vi "Execute (Multiple result with rows).vi"(8 "error in (no error)":errorcluster, 10 "SQL":string, 11 "PQ Connection in":refnum<class "PQ Connection.lvclass">) -> (0 "error out":errorcluster, 1 "Results with Rows returned":refnum<class "PQ Result.lvclass">[](array[class]), 3 "PQ Connection out":refnum<class "PQ Connection.lvclass">)   [LabVIEW 2016, in "PQ Connection.lvclass"]
uses:
  PQ Connection.lvclass
  Result/PQ Result.lvclass
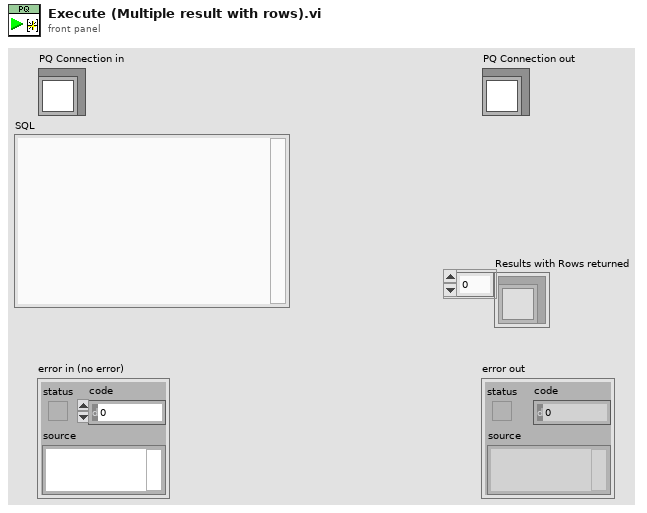
[diagram p1: front panel]
types:
  T1 = typedef "PQ Result.lvclass/Result Status.ctl" = enum32{"PGRES_EMPTY_QUERY", "PGRES_COMMAND_OK", "PGRES_TUPLES_OK", "PGRES_COPY_OUT", "PGRES_COPY_IN", "PGRES_BAD_RESPONSE", "PGRES_NONFATAL_ERROR", "PGRES_FATAL_ERROR", "PGRES_COPY_BOTH", "PGRES_SINGLE_TUPLE"}
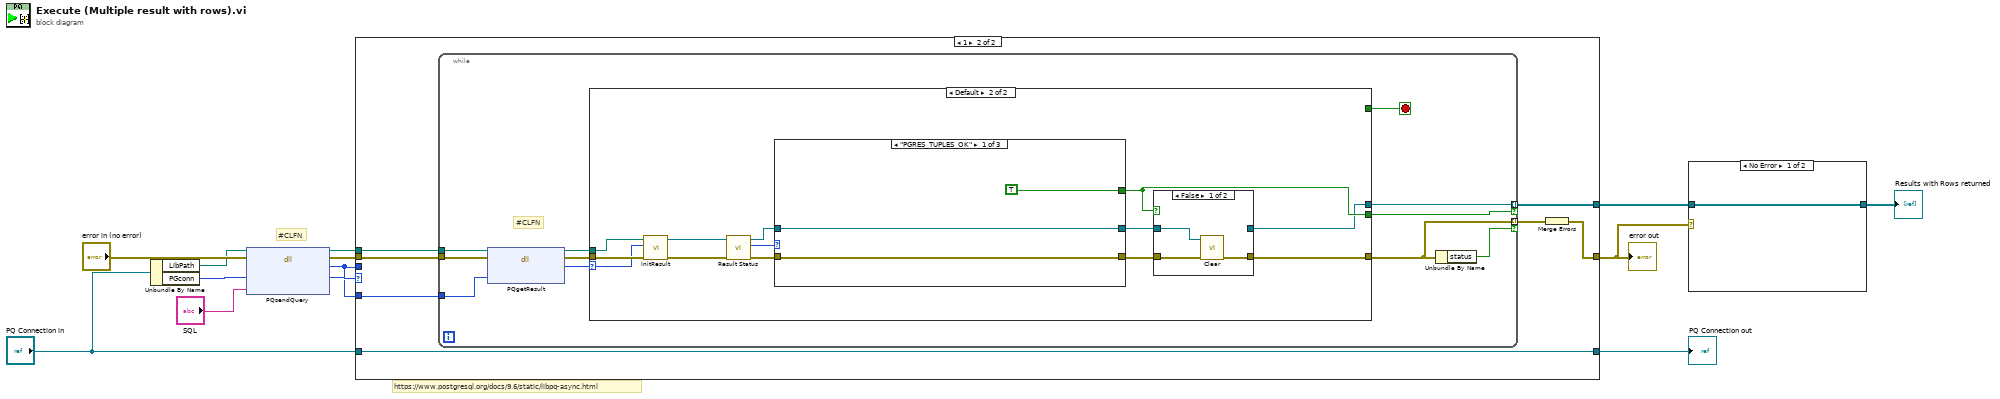
[diagram p0: block diagram]
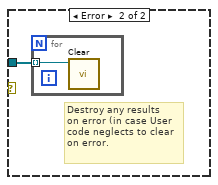
[diagram p2: hidden frame]
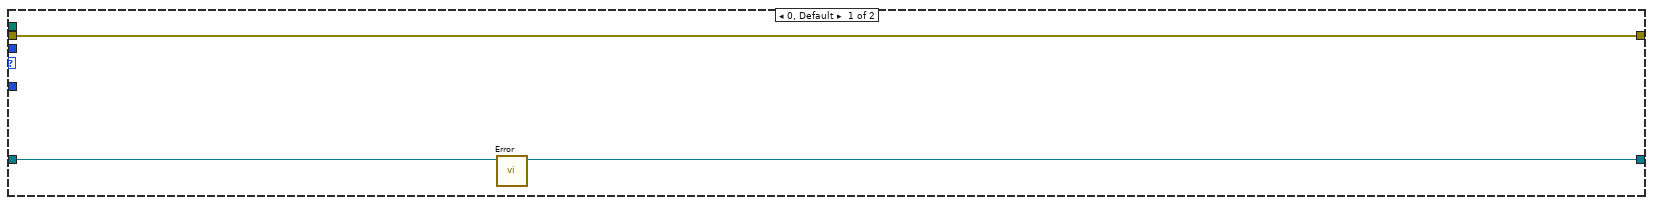
[diagram p3: hidden frame]
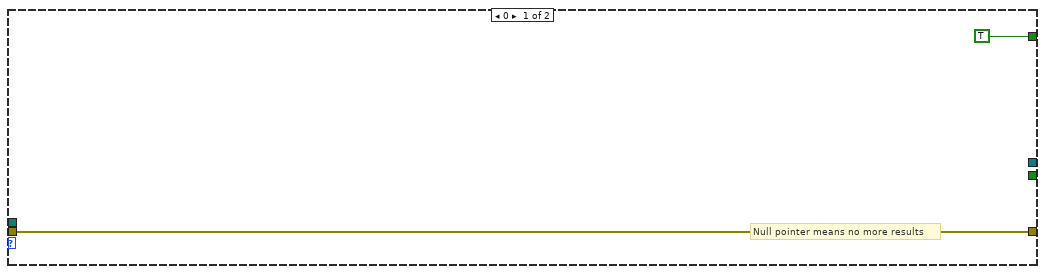
[diagram p4: hidden frame]
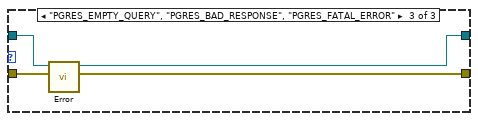
[diagram p6: hidden frame]
diagram:
  # "#CLFN"
  # "https://www.postgresql.org/docs/9.6/static/libpq-async.html"
  n1 = Unbundle By Name("PQ Connection in") -> ("LibPath"=w2:path, "PGconn"=w12:u32)
  n2 = dll-call lib="libpq.*" fn="PQsendQuery" ("libpq.*:PQexec")(path in=w2, error in="error in (no error)", "PGconn"=w12, "command"="SQL") -> (path out=w1:path, error out=w11:errorcluster, "OK?"=w9:u32, "PGconn"=w6:u32)  [unwired: 2 in]
  n3 = case shown="1" w9 {
    tunnel: w11 -> [w14 w23]
    tunnel: w9 -> [_ _]
    tunnel: [_ w22] -> w4
    tunnel: [w14 w18] -> w3
    tunnel: "PQ Connection in" -> [w16 w19]
    tunnel: [w15 w19] -> w7
    tunnel: w6 -> [_ w20]
    tunnel: w1 -> [_ w17]
    frame 0, Default {
      n4 = call "Error.vi"("PQ Connection in"=w16) -> ("PQ Connection out"=w15:refnum<class "PQ Connection.lvclass">)  [unwired: 9 in, 1 out]
    }
    frame 1 {
      n5 = while {
        tunnel: [w32] -> w22 mode=indexing if=w33
        tunnel: w20 -> [w34]
        tunnel: w23 -> [w29]
        tunnel: [w27] -> w21 mode=indexing if=w26
        tunnel: w17 -> [w25]
        stop <- w30 stop-if-true
        # "#CLFN"
        n6 = dll-call lib="libpq.*" fn="PQgetResult" ("libpq.*:PQexec")(path in=w25, error in=w29, "PGconn"=w34) -> (path out=w24:path, error out=w28:errorcluster, "PQresult"=w31:u32)  [unwired: 2 in]
        n7 = case shown="Default" w31 {
          selector: w31 -> [_ w39]
          tunnel: w28 -> [w36 w41]
          tunnel: [_ w49] -> w33
          tunnel: [_ w47] -> w32
          tunnel: [w36 w45] -> w27
          tunnel: [TRUE _] -> w30
          tunnel: w24 -> [_ w38]
          frame 0 {
            # "Null pointer means no more results"
          }
          frame Default {
            n8 = call "InitResult.vi"("error in (no error)"=w41, "PGresult"=w39, "LibPath"=w38) -> ("error out"=w40:errorcluster, "PQ Result out"=w37:refnum<class "PQ Result.lvclass">)  [unwired: 7 in]
            n9 = call "Result Status.vi"("error in (no error)"=w40, "PQ Result in"=w37) -> ("error out"=w42:errorcluster, "Result Status"=w44:T1, "PQ Result out"=w43:refnum<class "PQ Result.lvclass">)  [unwired: 7 in]
            n10 = case shown="\"PGRES_TUPLES_OK\"" w44 {
              tunnel: [w51 w53 w55] -> w48
              tunnel: w43 -> [w51 w53 w58]
              tunnel: w42 -> [w52 w54 w57]
              tunnel: [w52 w54 w56] -> w46
              tunnel: [TRUE _ _] -> w49
              frame "PGRES_TUPLES_OK" {
              }
              frame Default {
                # "No results, but not error"
              }
              frame "PGRES_EMPTY_QUERY", "PGRES_BAD_RESPONSE", "PGRES_FATAL_ERROR" {
                n11 = call "Error.vi"("error in (no error)"=w57, "PQ Result  In"=w58) -> ("error out"=w56:errorcluster, "PQ Result"=w55:refnum<class "PQ Result.lvclass">)  [unwired: 8 in]
              }
            }
            n12 = case shown="False" w49 {
              tunnel: w48 -> [w61 w63]
              tunnel: [_ w63] -> w47
              tunnel: w46 -> [w60 w62]
              tunnel: [w59 w62] -> w45
              frame False {
                n13 = call "Clear.vi"("error in (no error)"=w60, "PQ Result  in"=w61) -> ("error out"=w59:errorcluster)  [unwired: 9 in]
              }
              frame True {
              }
            }
          }
        }
        n14 = Unbundle By Name(w27) -> ("status"=w26:bool)
      }
      n15 = Merge Errors(w21) -> (w18:errorcluster)
    }
  }
  "error out" <- w3
  "PQ Connection out" <- w7
  n16 = case shown="No Error" w3 {
    tunnel: [w64 _] -> w5
    tunnel: w4 -> [w64 w65]
    frame No Error {
    }
    frame Error {
      # "Destroy any results\non error (in case User\ncode neglects to clear\non error."
      n17 = for {
        tunnel: w65 -> [w66] mode=indexing
        n18 = call "Clear.vi"("PQ Result  in"=w66) -> ()  [unwired: 10 in, 1 out]
      }
    }
  }
  "Results with Rows returned" <- w5
